vi "Initialize.vi"(8 "error in (no error)":errorcluster, 11 "handler in":refnum<class "Formatting Handler.lvclass">) -> (0 "error out":errorcluster, 3 "handler out":refnum<class "Formatting Handler.lvclass">)   [LabVIEW 2018, in "Logging.lvlib" / "Formatting Handler.lvclass"]
uses:
  Formatting Handler.lvclass
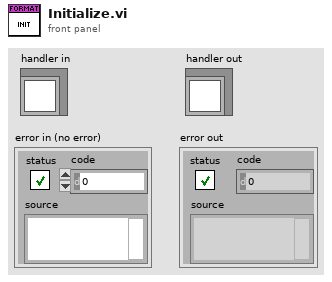
[diagram p1: front panel]
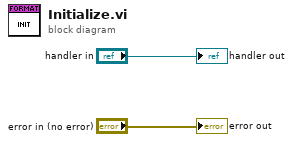
[diagram p0: block diagram]
diagram:
  "error out" <- "error in (no error)"
  "handler out" <- "handler in"
